vi "test Encapsulate.vi"(8 "error in (no error)":errorcluster, 11 "TestCase in":refnum<class "Lifecycle Tests.lvclass">) -> (0 "error out":errorcluster, 3 "TestCase out":refnum<class "Lifecycle Tests.lvclass">)   [LabVIEW 2017, in "Pointer Tests.lvlib" / "Lifecycle Tests.lvclass"]
uses:
  Lifecycle Tests.lvclass
  Source/Classes/Pointer/Public/New/New (4B).vi
  Source/Classes/Pointer/Public/Write/Write (1D I32).vi
  Source/Classes/Pointer/Public/Read/Read (0D I32).vi
  Source/Classes/Pointer/Public/Write/Write (0D I32).vi
  <vilib>/addons/_JKI Toolkits/VI Tester/TestCase.llb/TestCase.lvclass
  Source/Classes/Pointer/Pointer.lvclass
  C:/Program Files (x86)/National Instruments/LabVIEW 2017/vi.lib/addons/_JKI Toolkits/VI Tester/TestCase.llb/TestCase.lvclass
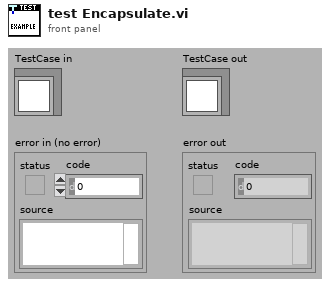
[diagram p1: front panel]
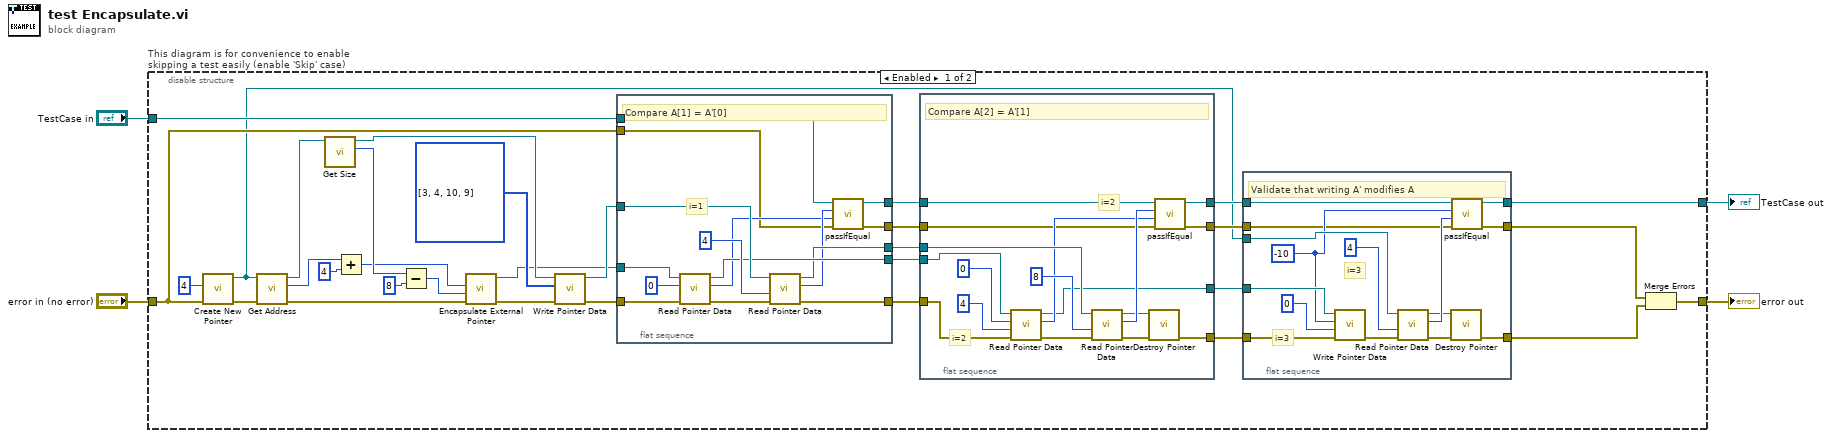
[diagram p0: block diagram]
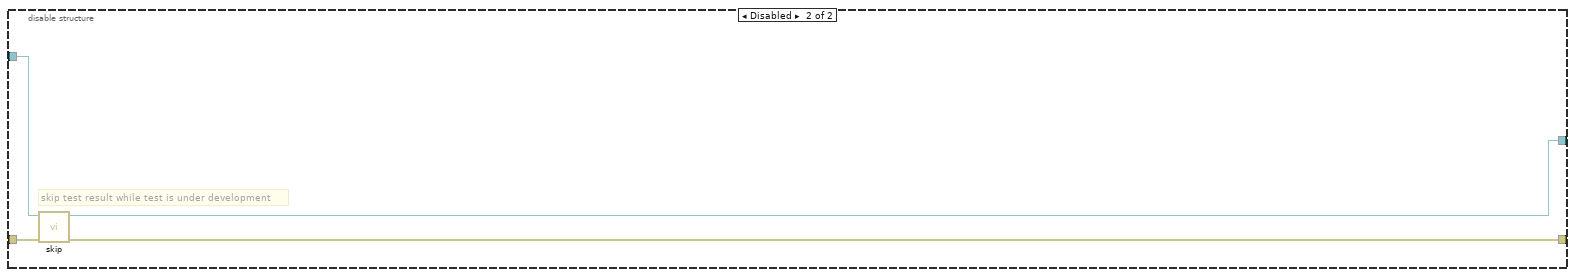
[diagram p2: hidden frame]
diagram:
  n1 = disable-structure "This diagram is for convenience to enable skipping a test easily (enable 'Skip' case)" shown="Enabled" {
    disable-tunnel: "TestCase in" -> [w10 w86]
    disable-tunnel: [w7 w84] -> w1
    disable-tunnel: [w20 w85] -> w3
    disable-tunnel: "error in (no error)" -> [w6 w83]
    frame Enabled {
      n2 = call-poly "Create New Pointer.vi"("error in (no error)"=w6, "count (1)"=u64 4) -> ("error out"=w28:errorcluster, "Pointer"=w5:refnum<class "Pointer.lvclass">)  [unwired: 8 in]
      n3 = call "Get Address.vi"("Pointer in"=w5) -> ("address"=w34:u64, "Pointer out"=w35:refnum<class "Pointer.lvclass">)  [unwired: 9 in]
      n4 = call "Get Size.vi"("Pointer in"=w35) -> ("size"=w32:u64, "Pointer out"=w27:refnum<class "Pointer.lvclass">)  [unwired: 9 in]
      n5 = Add(x=w34, y=u64 4) -> (x+y=w30:u64)
      n6 = Subtract(x=w32, y=u64 8) -> (x-y=w29:u64)
      n7 = call "Encapsulate External Pointer.vi"("error in (no error)"=w28, "size"=w29, "address"=w30) -> ("error out"=w26:errorcluster, "Pointer out"=w18:refnum<class "Pointer.lvclass">)  [unwired: 7 in]
      n8 = call-poly "Write Pointer Data.vi"("error in (no error)"=w26, "buffer in"=i32[] [3, 4, 10, 9] ("length (-1: rest)"), "Pointer in"=w27) -> ("error out"=w11:errorcluster, "Pointer out"=w24:refnum<class "Pointer.lvclass">)  [unwired: 5 in, 2 out]
      n9 = flat-sequence {
        tunnel: w24 -> [w82]
        tunnel: [w79] -> w23
        tunnel: [w78] -> w22
        tunnel: w18 -> [w75]
        tunnel: [w73] -> w17
        tunnel: [w72] -> w12
        tunnel: w11 -> [w71]
        tunnel: w10 -> [w70]
        tunnel: [w69] -> w9
        tunnel: w6 -> [w68]
        frame #0 {
          # "i=1"
          # "Compare A[1] = A'[0]"
          n10 = call-poly "Read Pointer Data.vi"("error in (no error)"=w71, "value in"=0 ("length (-1: rest)"), "Pointer in"=w75) -> ("error out"=w74:errorcluster, "value out"=w76:i32, "Pointer out"=w79:refnum<class "Pointer.lvclass">)  [unwired: 5 in, 1 out]
          n11 = call-poly "Read Pointer Data.vi"("error in (no error)"=w74, "offset (0)"=u64 4, "Pointer in"=w82) -> ("error out"=w72:errorcluster, "value out"=w77:i32, "Pointer out"=w78:refnum<class "Pointer.lvclass">)  [unwired: 5 in, 1 out]
          n12 = call-dynamic "passIfEqual.vi"("error in (no error)"=w68, "y"=w76, "x"=w77, "TestCase in"=w70) -> ("error out"=w73:errorcluster, "TestCase out"=w69:refnum<class "Lifecycle Tests.lvclass">)  [unwired: 6 in]
        }
      }
      n13 = flat-sequence {
        tunnel: w23 -> [w52]
        tunnel: w22 -> [w49]
        tunnel: [w45] -> w21
        tunnel: w17 -> [w43]
        tunnel: [w42] -> w16
        tunnel: [w37] -> w13
        tunnel: w12 -> [w40]
        tunnel: w9 -> [w39]
        tunnel: [w38] -> w8
        frame #0 {
          # "i=2"
          # "i=2"
          # "Compare A[2] = A'[1]"
          n14 = call-poly "Read Pointer Data.vi"("error in (no error)"=w40, "offset (0)"=u64 4, "value in"=0 ("length (-1: rest)"), "Pointer in"=w52) -> ("error out"=w44:errorcluster, "value out"=w46:i32, "Pointer out"=w45:refnum<class "Pointer.lvclass">)  [unwired: 4 in, 1 out]
          n15 = call-poly "Read Pointer Data.vi"("error in (no error)"=w44, "offset (0)"=u64 8, "Pointer in"=w49) -> ("error out"=w41:errorcluster, "value out"=w47:i32, "Pointer out"=w36:refnum<class "Pointer.lvclass">)  [unwired: 5 in, 1 out]
          n16 = call "Destroy Pointer.vi"("error in (no error)"=w41, "Pointer in"=w36) -> ("error out"=w37:errorcluster)  [unwired: 8 in, 1 out]
          n17 = call-dynamic "passIfEqual.vi"("error in (no error)"=w43, "y"=w46, "x"=w47, "TestCase in"=w39) -> ("error out"=w42:errorcluster, "TestCase out"=w38:refnum<class "Lifecycle Tests.lvclass">)  [unwired: 6 in]
        }
      }
      n18 = flat-sequence {
        tunnel: w21 -> [w67]
        tunnel: w5 -> [w66]
        tunnel: w16 -> [w61]
        tunnel: [w60] -> w15
        tunnel: [w54] -> w14
        tunnel: w13 -> [w58]
        tunnel: w8 -> [w57]
        tunnel: [w56] -> w7
        frame #0 {
          w65 = -10 ("length (-1: rest)")
          # "i=3"
          # "i=3"
          # "Validate that writing A' modifies A"
          n19 = call-poly "Write Pointer Data.vi"("error in (no error)"=w58, "offset (0)"=u64 0, "value"=w65, "Pointer in"=w67) -> ("error out"=w62:errorcluster)  [unwired: 4 in, 3 out]
          n20 = call-poly "Read Pointer Data.vi"("error in (no error)"=w62, "offset (0)"=u64 4, "Pointer in"=w66) -> ("error out"=w59:errorcluster, "value out"=w63:i32, "Pointer out"=w53:refnum<class "Pointer.lvclass">)  [unwired: 5 in, 1 out]
          n21 = call "Destroy Pointer.vi"("error in (no error)"=w59, "Pointer in"=w53) -> ("error out"=w54:errorcluster)  [unwired: 8 in, 1 out]
          n22 = call-dynamic "passIfEqual.vi"("error in (no error)"=w61, "y"=w63, "x"=w65, "TestCase in"=w57) -> ("error out"=w60:errorcluster, "TestCase out"=w56:refnum<class "Lifecycle Tests.lvclass">)  [unwired: 6 in]
        }
      }
      n23 = Merge Errors(w15, w14) -> (w20:errorcluster)
    }
    frame Disabled {
      # "skip test result while test is under development"
      n24 = call <vilib>:"skip.vi"("error in (no error)"=w83, "TestCase in"=w86) -> ("error out"=w85:errorcluster, "TestCase out"=w84:refnum<class "Lifecycle Tests.lvclass">)  [unwired: 8 in]
    }
  }
  "error out" <- w3
  "TestCase out" <- w1
